vi "SENS_CORR_COLL_GUID_CONN_CAT.vi"(0 "VISA IN":refnum<visa-resource-name>, 5 "error in":errorcluster, 7 "Channel":i32) -> (14 "VISA Out":refnum<visa-resource-name>, 17 "ConnType":string[](array[string]), 19 "error out":errorcluster)   [LabVIEW 2018, in "PNA-X.lvlib"]
doc: "SENSe<cnum>:FOM:CATalog? \n(Read-only) Returns a comma-separated list of available range names in the PNA. \nParameters \n<cnum> Any existing channel number; if unspecified, value is set to 1. \nExamples SENS:FOM:CAT? \n'returns \n\"Primary, Source, Receivers\" \nReturn Type String \nDefault Not Applicable"
uses:
  PNA-X.lvlib
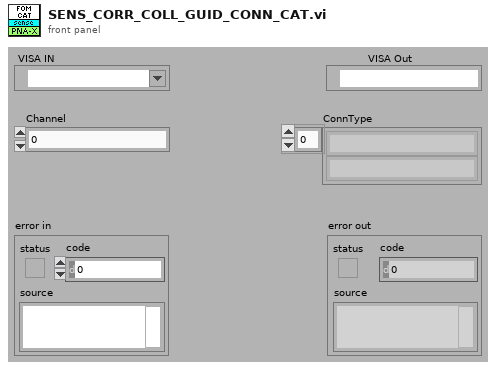
[diagram p1: front panel]
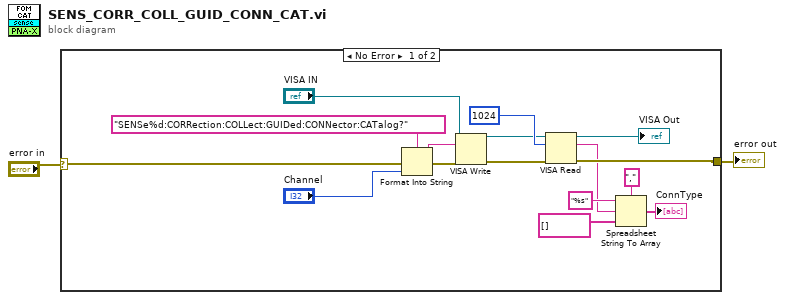
[diagram p0: block diagram]
diagram:
  n1 = case shown="No Error" "error in" {
    selector: "error in" -> [w18 w19]
    tunnel: [w9 w19] -> w1
    frame No Error {
      n2 = Format Into String(format string="SENSe%d:CORRection:COLLect:GUIDed:CONNector:CATalog?" ("Cmdline"), error in=w18, "Channel") -> (resulting string=w16:string, error out=w17:errorcluster)  [unwired: 1 in]
      n3 = VISA Write(VISA resource name="VISA IN", write buffer=w16, error in (no error)=w17) -> (VISA resource name out=w11:refnum<visa-resource-name>, error out=w13:errorcluster)  [unwired: 1 out]
      n4 = VISA Read(VISA resource name=w11, byte count=1024, error in (no error)=w13) -> (VISA resource name out=→"VISA Out":refnum<visa-resource-name>, read buffer=w4:string, error out=w9:errorcluster)  [unwired: 1 out]
      n5 = Spreadsheet String To Array(delimiter (Tab)=",", format string="%s", spreadsheet string=w4, array type (2D Dbl)=string[] []) -> (array=→"ConnType":string[])
    }
    frame Error {
    }
  }
  "error out" <- w1
